vi "Generator High Speed PIDDW.vi"() -> ()   [LabVIEW 2019]
uses:
  <vilib>/Instr/_visa.llb/VISA Configure Serial Port (Instr).vi
panel:
  in  "Wave Off":dbl(slide)=331.63265306122446 scale=0.0..500.0
  in  "Square":bool
  in  "Auto":bool=TRUE
  in  "Amp":dbl(slide)=153.0612244897959 scale=0.0..500.0
  in  "Wave Per":dbl(slide)=255.10204081632654 scale=0.0..100.0
  in  "ReInit":bool
  in  "Output Limits":cluster{"Hi":dbl, "Low":dbl}={"Hi"=255.0, "Low"=-255.0}
  in  "PID Coefficients":cluster{"P":dbl, "I":dbl, "D":dbl}={"P"=0.05, "I"=5.0, "D"=0.0}
  out "Output":u8=109
  out "Error":i16=16
  out "mWatts":sgl=-0.83192945 format="%#_3g"
  out "Freq. Hz":dbl=43.47826086956522 format="%#_3g"
  out "dt out (s)":dbl=0.023 format="%.3f"
  in  "Loop Per":dbl(slide)=22.95918367346939 scale=0.0..50.0
  in  "V Setpoint":i16(slide)=143 scale=0.0..1000.0
  in  "Load Level":u8(slide) scale=0.0..40.0
  in  "stop":bool
  out "Waveform Chart":cluster{"V Setpoint":dbl, i16}(graph)={"V Setpoint"=484.69387755102036, 469}
  in  "Baud Rate (9600)":u32=115200
  in  "VISA resource name":refnum<visa-resource-name>="COM28"
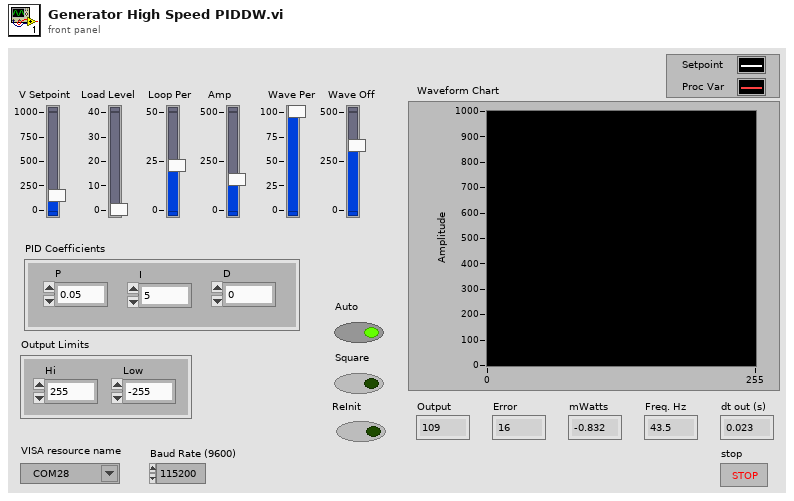
[diagram p1: front panel]
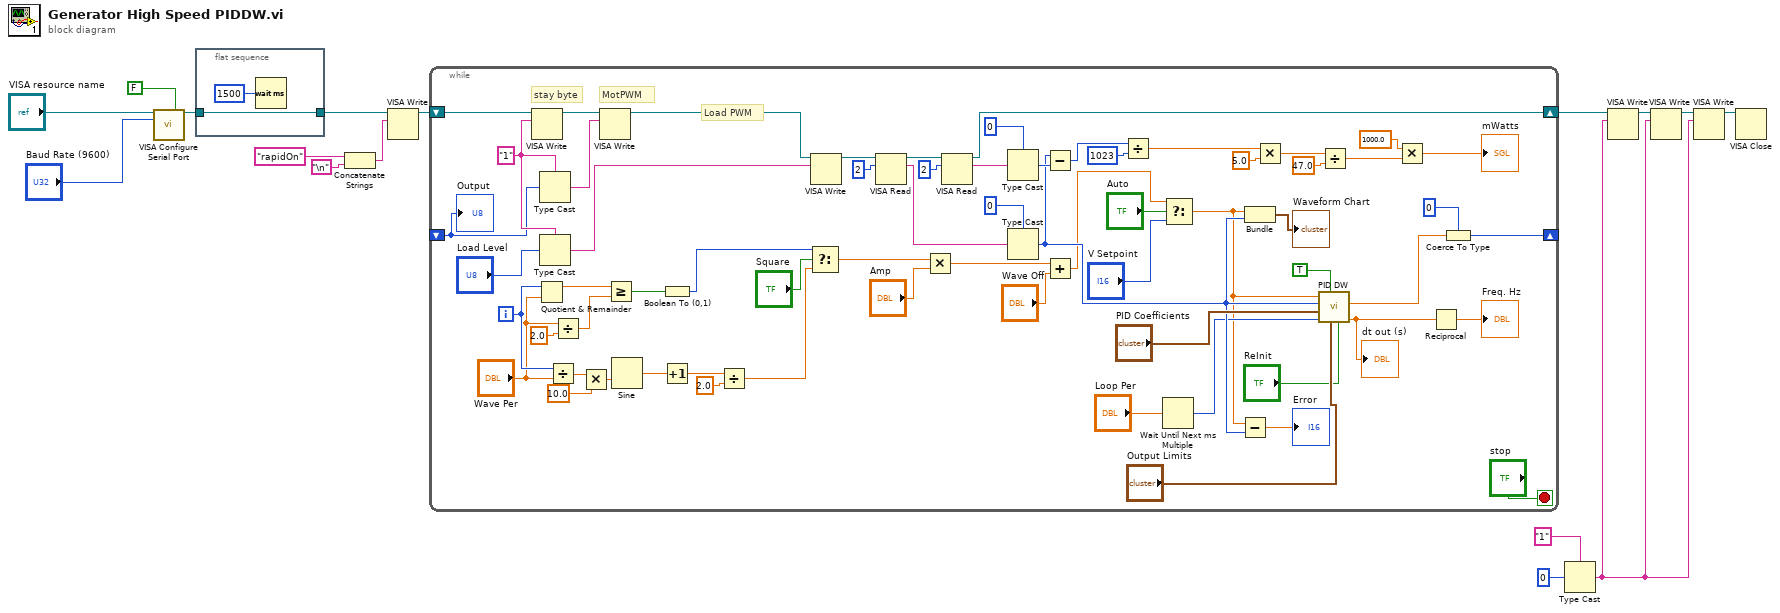
[diagram p0: block diagram]
diagram:
  n1 = call-poly "VISA Configure Serial Port"("VISA resource name"="VISA resource name", "Enable Termination\nChar (T)"=FALSE ("Enable Termination\nChar (T)"), "baud rate (9600)"="Baud Rate (9600)") -> ("VISA resource name out"=w11:refnum<visa-resource-name>)  [unwired: 11 in, 1 out]
  n2 = flat-sequence {
    tunnel: w11 -> [w17]
    tunnel: [w17] -> w10
    frame #0 {
      n3 = Wait (ms)(milliseconds to wait=u32 1500) -> ()  [unwired: 1 out]
    }
  }
  n4 = Concatenate Strings("rapidOn" ("string"), "\n") -> (w14:string)
  n5 = VISA Write(VISA resource name=w10, write buffer=w14) -> (VISA resource name out=w9:refnum<visa-resource-name>)  [unwired: 1 in, 2 out]
  n6 = while {
    shift-right: [w65] -> w5
    shift-left: w9 -> [w83]
    shift-right: [w68] -> _
    shift-left: _ -> [w71]
    i -> [w23]
    stop <- "stop" stop-if-true
    w72 = "1"
    # "Load PWM"
    # "MotPWM"
    # "stay byte"
    n7 = VISA Write(VISA resource name=w83, write buffer=w72) -> (VISA resource name out=w78:refnum<visa-resource-name>)  [unwired: 1 in, 2 out]
    n8 = Quotient & Remainder(x=w23, y="Wave Per") -> (x-y*floor(x/y)=w37:dbl)  [unwired: 1 out]
    n9 = Type Cast(type=w72, x=w71) -> (*(type *) &x=w75:string)
    n10 = Type Cast(type=w72, x="Load Level") -> (*(type *) &x=w73:string)
    n11 = Divide(x=w23, y="Wave Per") -> (x/y=w21:dbl)
    n12 = Divide(x="Wave Per", y=2.0) -> (x/y=w36:dbl)
    n13 = Multiply(x=w21, y=10.0) -> (x*y=w19:dbl)
    n14 = VISA Write(VISA resource name=w78, write buffer=w75) -> (VISA resource name out=w81:refnum<visa-resource-name>)  [unwired: 1 in, 2 out]
    n15 = Greater Or Equal?(x=w37, y=w36) -> (x >= y?=w35:bool)
    n16 = Sine(x=w19) -> (sin(x)=w30:dbl)
    n17 = Boolean To (0,1)(Boolean=w35) -> (0, 1=w27:i16)
    n18 = Increment(x=w30) -> (x+1=w29:dbl)
    n19 = Divide(x=w29, y=2.0) -> (x/y=w26:dbl)
    n20 = Select(t=w27, s="Square", f=w26) -> (s? t:f=w25:dbl)
    n21 = VISA Write(VISA resource name=w81, write buffer=w73) -> (VISA resource name out=w80:refnum<visa-resource-name>)  [unwired: 1 in, 2 out]
    n22 = VISA Read(VISA resource name=w80, byte count=u32 2) -> (VISA resource name out=w66:refnum<visa-resource-name>, read buffer=w77:string)  [unwired: 1 in, 2 out]
    n23 = Multiply(x=w25, y="Amp") -> (x*y=w33:dbl)
    n24 = VISA Read(VISA resource name=w66, byte count=u32 2) -> (VISA resource name out=w65:refnum<visa-resource-name>, read buffer=w63:string)  [unwired: 1 in, 2 out]
    n25 = Type Cast(type=i16 0, x=w63) -> (*(type *) &x=w62:i16)
    n26 = Type Cast(type=i16 0, x=w77) -> (*(type *) &x=w46:i16)
    n27 = Subtract(x=w46, y=w62) -> (x-y=w58:i16)
    n28 = Add(x=w33, y="Wave Off") -> (x+y=w31:dbl)
    n29 = Divide(x=w58, y=i16 1023) -> (x/y=w56:dbl)
    n30 = Wait Until Next ms Multiple(millisecond multiple="Loop Per") -> (millisecond timer value=w42:u32)
    n31 = Select(t=w31, s="Auto", f="V Setpoint") -> (s? t:f=w40:dbl)
    n32 = Subtract(x=w40, y=w46) -> (x-y=→"Error":dbl)
    n33 = Bundle("V Setpoint"=w40, w46) -> (→"Waveform Chart":cluster{"V Setpoint":dbl, i16})  [unwired: 1 in]
    n34 = Multiply(x=w56, y=5.0) -> (x*y=w54:dbl)
    n35 = call "PID DW.vi"("Init?"="ReInit", "Output Limits"="Output Limits", "Auto/Manual"=TRUE, "dT(in)"=w42, "PID Coefficients"="PID Coefficients", "Process Variable"=w46, "Setpoint"=w40) -> ("dT"=w43:dbl, "Output"=w51:dbl)  [unwired: 3 in]
    "dt out (s)" <- w43
    n36 = Divide(x=w54, y=sgl 47.0) -> (x/y=w60:dbl)
    n37 = Multiply(x=1000.0, y=w60) -> (x*y=→"mWatts":dbl)
    n38 = Reciprocal(x=w43) -> (1/x=→"Freq. Hz":dbl)
    n39 = Coerce To Type(0:w51, 1:u8 0) -> (2:w68:u8)
    "Output" <- w71
  }
  n40 = Type Cast(type="1", x=u32 0 ("millisecond multiple")) -> (*(type *) &x=w3:string)
  n41 = VISA Write(VISA resource name=w5, write buffer=w3) -> (VISA resource name out=w6:refnum<visa-resource-name>)  [unwired: 1 in, 2 out]
  n42 = VISA Write(VISA resource name=w6, write buffer=w3) -> (VISA resource name out=w7:refnum<visa-resource-name>)  [unwired: 1 in, 2 out]
  n43 = VISA Write(VISA resource name=w7, write buffer=w3) -> (VISA resource name out=w4:refnum<visa-resource-name>)  [unwired: 1 in, 2 out]
  n44 = VISA Close(VISA resource name=w4) -> ()  [unwired: 1 in, 1 out]
